vi "Add Suffix to Topology.vi"(8 "topology suffix":string, 10 "Topology in":T1) -> (1 "Topology out":T1)   [LabVIEW 2016, in "SLSC Switch.lvlib" / "SLSC Switch.lvclass"]
uses:
  SLSC Switch.lvclass
  Controls/Topology.ctl
  Controls/JSON.InitialState.ctl
  Controls/JSON.ChannelList.ctl
  Controls/JSON.ConnectionList.ctl
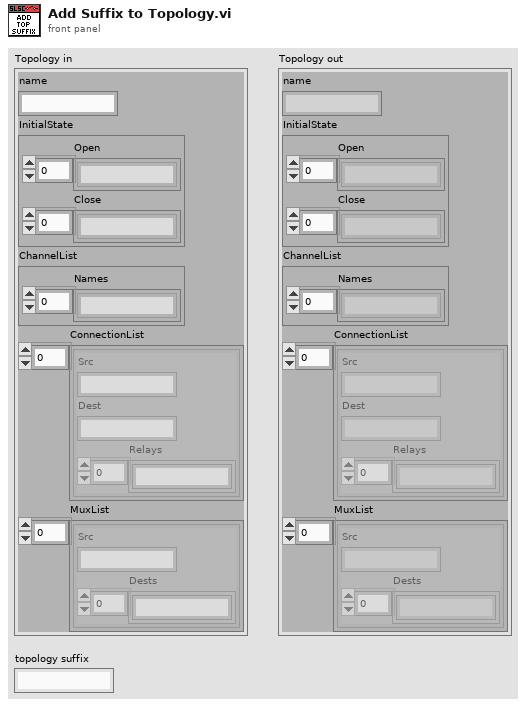
[diagram p1: front panel]
types:
  T1 = typedef "SLSC Switch.lvlib/SLSC Switch.lvclass/Topology.ctl" = cluster{"name":string, "InitialState":T2, "ChannelList":T3, "ConnectionList":T4[], "MuxList":cluster{"Src":string, "Dests":string[]}[]}
  T2 = typedef "SLSC Switch.lvlib/SLSC Switch.lvclass/JSON.InitialState.ctl" = cluster{"Open":string[], "Close":string[]}
  T3 = typedef "SLSC Switch.lvlib/SLSC Switch.lvclass/JSON.ChannelList.ctl" = cluster{"Names":string[]}
  T4 = typedef "SLSC Switch.lvlib/SLSC Switch.lvclass/JSON.ConnectionList.ctl" = cluster{"Src":string, "Dest":string, "Relays":string[]}
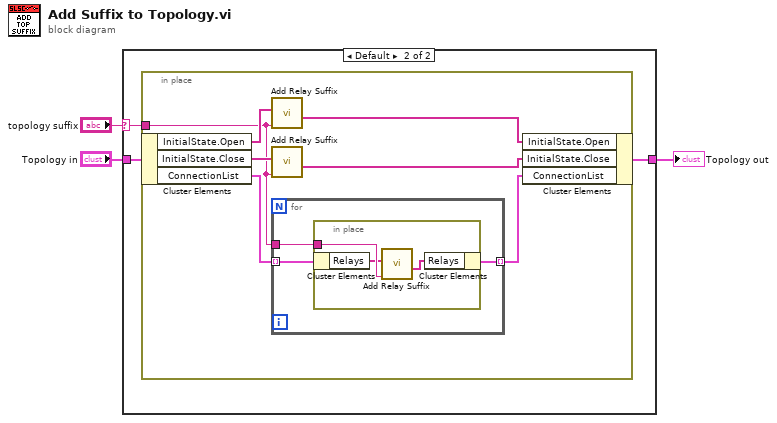
[diagram p0: block diagram]
diagram:
  n1 = case shown="Default" "topology suffix" {
    selector: "topology suffix" -> [_ w7]
    tunnel: [w4 w6] -> w2
    tunnel: "Topology in" -> [w4 w5]
    frame "" {
    }
    frame Default {
      n2 = in-place {
        in-place-border: w7 -> [w9]
        n3 = in-place-cluster #1(w5) -> ("InitialState.Open"=w11:string[], "InitialState.Close"=w10:string[], "ConnectionList"=w14:T4[])
        n4 = call "Add Relay Suffix.vi"("topology suffix"=w9, "Relays"=w11) -> ("Array"=w12:string[])  [unwired: 9 in]
        n5 = call "Add Relay Suffix.vi"("topology suffix"=w9, "Relays"=w10) -> ("Array"=w8:string[])  [unwired: 9 in]
        n6 = for {
          tunnel: w14 -> [w17] mode=indexing
          tunnel: [w16] -> w13 mode=indexing
          tunnel: w9 -> [w15]
          n7 = in-place {
            in-place-border: w15 -> [w20]
            n8 = in-place-cluster #2(w17) -> ("Relays"=w19:string[])
            n9 = call "Add Relay Suffix.vi"("topology suffix"=w20, "Relays"=w19) -> ("Array"=w18:string[])  [unwired: 9 in]
            n10 = in-place-cluster #2("Relays"=w18) -> (w16:T4)
          }
        }
        n11 = in-place-cluster #1("InitialState.Open"=w12, "InitialState.Close"=w8, "ConnectionList"=w13) -> (w6:T1)
      }
    }
  }
  "Topology out" <- w2
